vi "avToULong64Image.vi"(5 "attribute value":T1={"device name"="", "attribute name"="", "quality value"=0, "quality string"="", "timestamp"=0.0, "dim. x"=0, "dim. y"=0, "value"=[], "error code"=0, "error stack"=[], "data type"=36}) -> (0 "value":u32[][](array[numeric]), 1 "quality":i16, 2 "attribute name":string, 3 "device name":string, 4 "setpoint":u32[][](array[numeric]))   [LabVIEW 2014, in "tango.lvlib"]
uses:
  tango.lvlib
  base/toULong64Image.vi
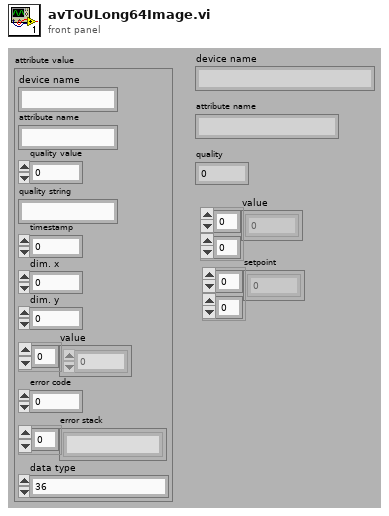
[diagram p1: front panel]
types:
  T1 = cluster{"device name":string, "attribute name":string, "quality value":i16, "quality string":string, "timestamp":dbl, "dim. x":i32, "dim. y":i32, "value":u8[], "error code":i32, "error stack":string[], "data type":u16}
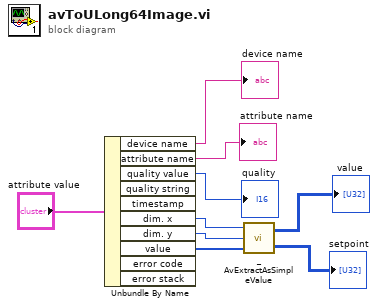
[diagram p0: block diagram]
diagram:
  n1 = Unbundle By Name("attribute value") -> ("device name"=→"device name":string, "attribute name"=→"attribute name":string, "quality value"=→"quality":i16, "dim. x"=w6:i32, "dim. y"=w7:i32, "value"=w8:u8[])  [unwired: 4 out]
  n2 = call-poly "_AvExtractAsSimpleValue.vi"("value_in"=w8, "dim_y"=w7, "dim_x"=w6) -> ("setpoint"=→"setpoint":u64[][], "value"=→"value":u64[][])
